vi "PID_18.06.vi"() -> ()   [LabVIEW 2017]
uses:
  <vilib>/Platform/TimedLoop/XDataNode/timing_clust.ctl
  <vilib>/Platform/TimedLoop/XDataNode/nitl_modes.ctl
  <vilib>/Platform/TimedLoop/XDataNode/wakeup.ctl
  <vilib>/platform/TimedLoop/XDataNode/XDataNode.xnode
  <vilib>/Platform/TimedLoop/XDataNode/XDNodeRunTimeDep.lvlib
panel:
  out "Period":i64
  out "Finished Late? [i-1]":bool
  out "Actual Start [i]":i64
  in  "PWM[%]":dbl(knob) scale=0.0..100.0
  in  "stop 2":bool
  in  "IP address":string
  out "Gauge":dbl(knob) scale=0.0..6000.0
  in  "stop":bool
  out "String":string
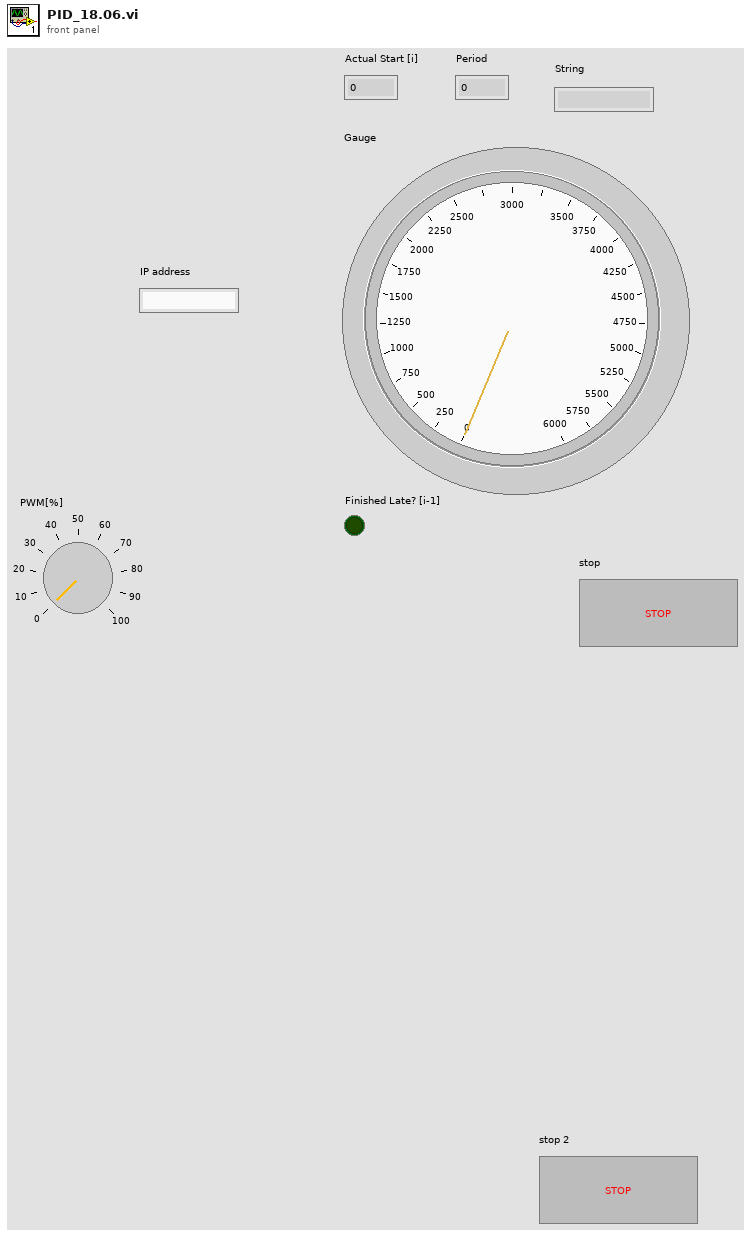
[diagram p1: front panel]
types:
  T1 = typedef "XDNodeRunTimeDep.lvlib/timing_clust.ctl" = cluster{"Expected End [f-1]":u64, "Actual End [f-1]":u64, "Finished Late? [f-1]":bool, "Expected End [i-1]":u64, "Actual End [i-1]":u64, "Finished Late? [i-1]":bool, "Expected Start [i]":u64, "Actual Start [i]":u64, "Expected Start [f]":u64, "Actual Start [f]":u64, "Source Name":string, "Structure Name":string, "Period":i64, "Deadline":i64, "Offset":i64, "Start":i64, "Priority":i32, "Timeout":i32, "Mode":T2, "Wakeup Reason":T3, "Error":errorcluster, "Source Type":string, "Secondary Source Type":string, "Global End Time":u64, "Global Start Time":u64, "Frame Duration":u64, "Iteration Duration":u64, "Assigned CPU":i32, "I/O Scan Engine Mode":u32}
  T2 = typedef "XDNodeRunTimeDep.lvlib/nitl_modes.ctl" = enum32{"No Change", "Process missed periods, maintain original phase", "Discard missed periods, maintain original phase", "Process missed periods, ignore original phase", "Discard missed periods, ignore original phase"}
  T3 = typedef "XDNodeRunTimeDep.lvlib/wakeup.ctl" = enum32{"Normal", "Aborted", "Asynchronous wakeup", "Timing source error", "Timed loop error", "Timeout"}
  T4 = enum16{"Standard", "Buffered", "CRLF", "Immediate"}
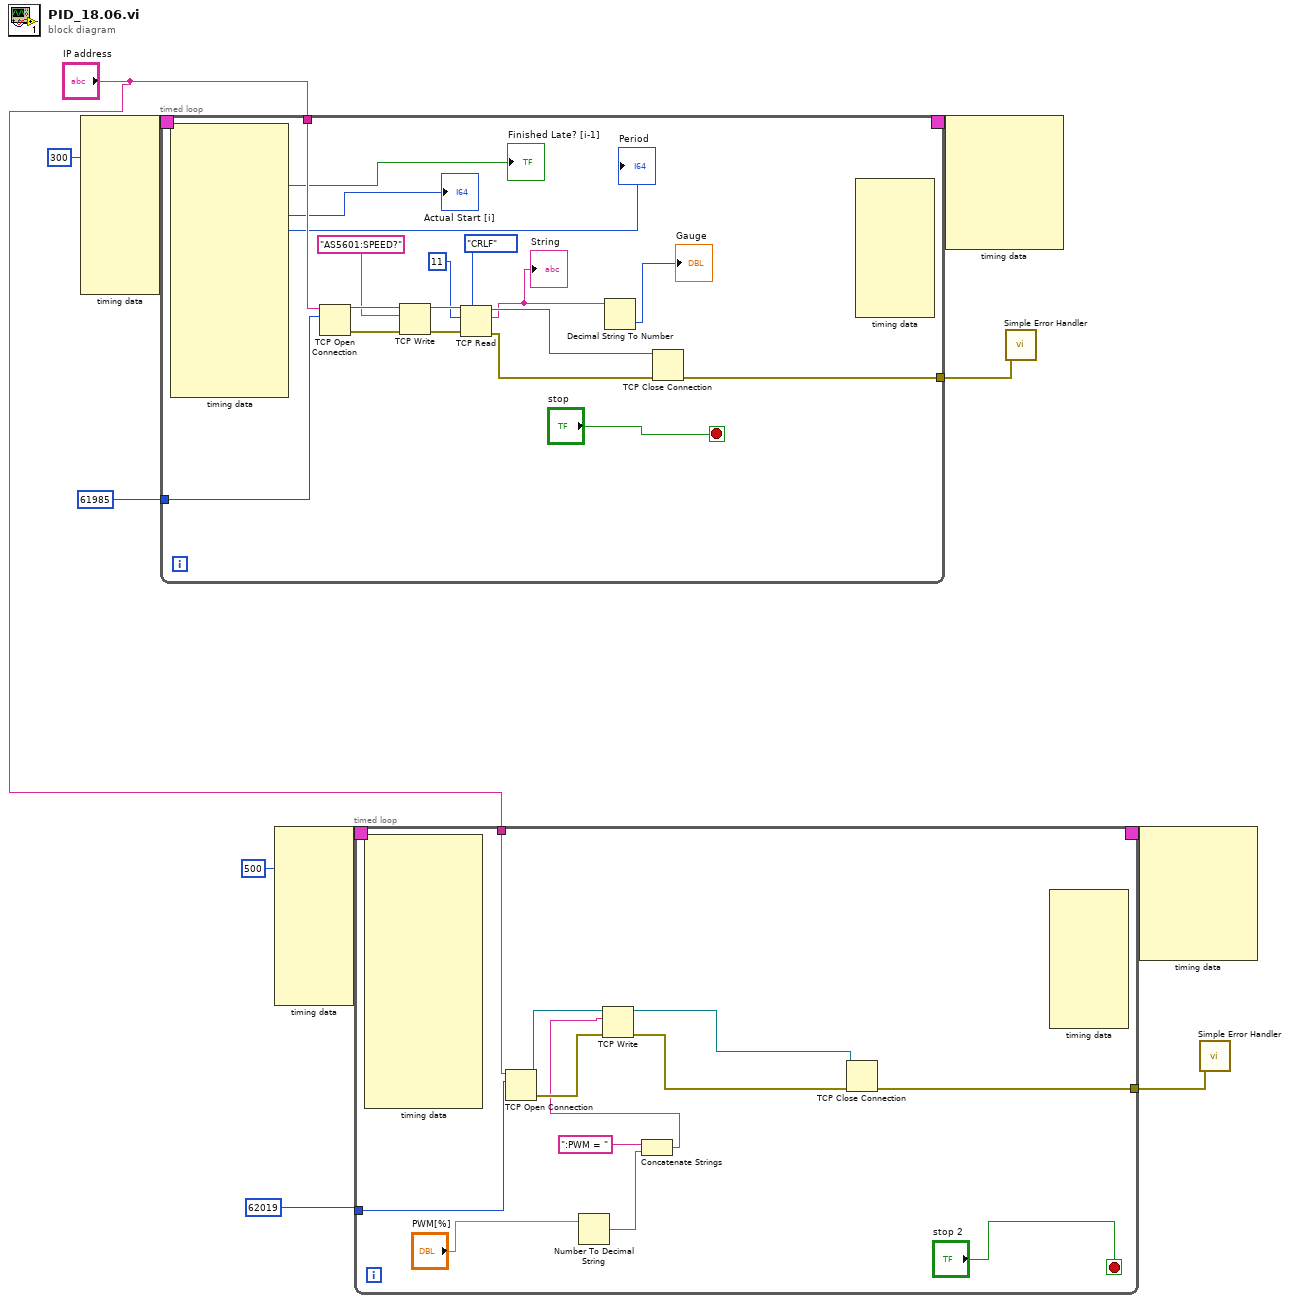
[diagram p0: block diagram]
diagram:
  n1 = node-c288(i64 300 ("Period")) -> (w10:T1)  [unwired: 9 in]
  n2 = timed-loop {
    tunnel: u16 61985 ("remote port\n or service name") -> [w25]
    tunnel: "IP address" -> [w24]
    tunnel: [w19] -> w11
    timing: w10 -> [_]
    timing-out: [_] -> w9
    stop <- "stop" stop-if-true
    n3 = node-c288() -> (→"Finished Late? [i-1]":bool, →"Actual Start [i]":i64, →"Period":i64)  [unwired: 1 in, 14 out]
    n4 = TCP Open Connection(address=w24, remote port or service name=w25) -> (connection ID=w22:refnum<k5>, error out=w23:errorcluster)  [unwired: 3 in]
    n5 = TCP Write(connection ID=w22, data in="AS5601:SPEED?", error in (no error)=w23) -> (connection ID out=w29:refnum<k5>, error out=w26:errorcluster)  [unwired: 1 in, 1 out]
    n6 = TCP Read(connection ID=w29, bytes to read=11, error in (no error)=w26, 7:T4."CRLF" ("mode (standard)")) -> (connection ID out=w20:refnum<k5>, data out=w17:string, error out=w21:errorcluster)  [unwired: 1 in]
    "String" <- w17
    n7 = Decimal String To Number(string=w17) -> (number=→"Gauge":i32)  [unwired: 2 in, 1 out]
    n8 = TCP Close Connection(connection ID=w20, error in (no error)=w21) -> (error out=w19:errorcluster)  [unwired: 1 in, 1 out]
    n9 = node-c288() -> ()  [unwired: 8 in, 1 out]
  }
  n10 = node-c288(i64 500 ("Period")) -> (w8:T1)  [unwired: 9 in]
  n11 = timed-loop {
    tunnel: u16 62019 ("remote port\n or service name 2") -> [w45]
    tunnel: "IP address" -> [w44]
    tunnel: [w41] -> w6
    timing: w8 -> [_]
    timing-out: [_] -> w7
    stop <- "stop 2" stop-if-true
    n12 = node-c288() -> ()  [unwired: 1 in, 17 out]
    n13 = TCP Open Connection(address=w44, remote port or service name=w45) -> (connection ID=w42:refnum<k5>, error out=w43:errorcluster)  [unwired: 3 in]
    n14 = Number To Decimal String(number="PWM[%]") -> (decimal integer string=w38:string)  [unwired: 1 in]
    n15 = Concatenate Strings(":PWM = ", w38) -> (w36:string)
    n16 = TCP Write(connection ID=w42, data in=w36, error in (no error)=w43) -> (connection ID out=w40:refnum<k5>, error out=w39:errorcluster)  [unwired: 1 in, 1 out]
    n17 = TCP Close Connection(connection ID=w40, error in (no error)=w39) -> (error out=w41:errorcluster)  [unwired: 1 in, 1 out]
    n18 = node-c288() -> ()  [unwired: 8 in, 1 out]
  }
  n19 = node-c288(w9) -> ()  [unwired: 7 out]
  n20 = call <vilib>:"Simple Error Handler.vi"("error in (no error)"=w11) -> ()  [unwired: 4 in, 5 out]
  n21 = node-c288(w7) -> ()  [unwired: 7 out]
  n22 = call <vilib>:"Simple Error Handler.vi"("error in (no error)"=w6) -> ()  [unwired: 4 in, 5 out]
